vi "10-1 GPIB driver one meas sol.vi"(4 "Function (0:V DC)":u16(ring) items=["DC Voltage", "AC Voltage", "2--Wire Resistance", "4-Wire Resistance", "DC Current", "AC Current", "Frequency", "Period", "Continuity", "Diode Checking", "VDC: VDC Ratio"], 7 "IDENTIF":bool, 8 "Manual Range (10.00)":dbl=7.0 min=0.0 format="%.2f", 9 "error in (no error)":errorcluster) -> (1 "Data value":dbl[](array[numeric]) format="%.4e", 6 "error out":errorcluster)   [LabVIEW 2012]
doc: "© Copyright M. Ferrari 2003\nMisura singola con HP34401A \nDRV per interfaccia GPIB"
uses:
  <instrlib>/Agilent 34401/Public/Data/Read (Single Point).vi
  <instrlib>/Agilent 34401/Agilent 34401.lvlib
panel:
  out "Measurement":dbl
  in  "VISA resource name":refnum<visa-resource-name>
  # "MISURA CON MULTIMETRO HP34401A ed USO dei VI del DRIVER di LabVIEW \n    Realizzare un VI che svolga le seguenti funzioni indicate utilizzando il driver contenuto\n    nella libreria degli strumenti e l'interfaccia HPIB :\n   - configura il multimetro per una misura di tensione continua su un range da 0 a 8V,\n     modificabile manualmente da pannello\n   - tramite un controllo booleano permette di abilitare o meno l'identificazione dello strumento\n     e verifica che si tratti del multimetro sopra indicato   \n   - esegue la misura, visualizza il valore letto e segnala gli eventuali errori"
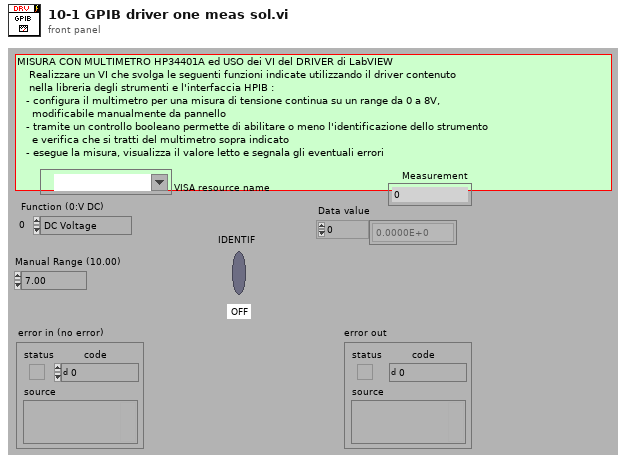
[diagram p1: front panel]
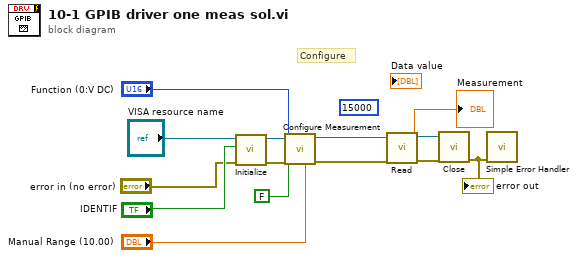
[diagram p0: block diagram]
diagram:
  (unwired) u32 15000 ("Timeout (60000 ms)")
  # "Configure"
  n1 = call <instrlib>:"Initialize.vi"("error in (no error)"="error in (no error)", "ID Query (True)"="IDENTIF", "VISA resource name"="VISA resource name") -> ("error out"=w12:errorcluster, "VISA resource name out"=w13:refnum<visa-resource-name>)  [unwired: 7 in]
  n2 = call <instrlib>:"Configure Measurement.vi"("Manual Range (1.00)"="Manual Range (10.00)", "error in (no error)"=w12, "Enable Auto Range (T: Enable)"=FALSE ("Range/Resolution (T:Auto)"), "Function (0: DC Voltage)"="Function (0:V DC)", "VISA resource name"=w13) -> ("error out"=w1:errorcluster, "VISA resource name out"=w2:refnum<visa-resource-name>)  [unwired: 5 in]
  n3 = call-poly <instrlib>:"Read.vi"("error in (no error)"=w1, "VISA resource name"=w2) -> ("error out"=w8:errorcluster, "Measurement"=→"Measurement":dbl, "VISA resource name out"=w7:refnum<visa-resource-name>)  [unwired: 7 in]
  n4 = call <instrlib>:"Close.vi"("error in (no error)"=w8, "VISA resource name"=w7) -> ("error out"=w6:errorcluster)  [unwired: 9 in]
  "error out" <- w6
  n5 = call <vilib>:"Simple Error Handler.vi"("error in (no error)"=w6) -> ()  [unwired: 4 in, 5 out]
